vi "OP30 Indicators.vi"(8 "error in (no error)":errorcluster, 10 "Array":refnum<vi>[](array[refnum]), 11 "OUTPUT INDICATOR in":T1) -> (0 "error out":errorcluster, 3 "OUTPUT INDICATOR out":T1)   [LabVIEW 2017]
uses:
  f95f8c13-f30c-4ba5-8700-8ca84cf3f7c2.vi
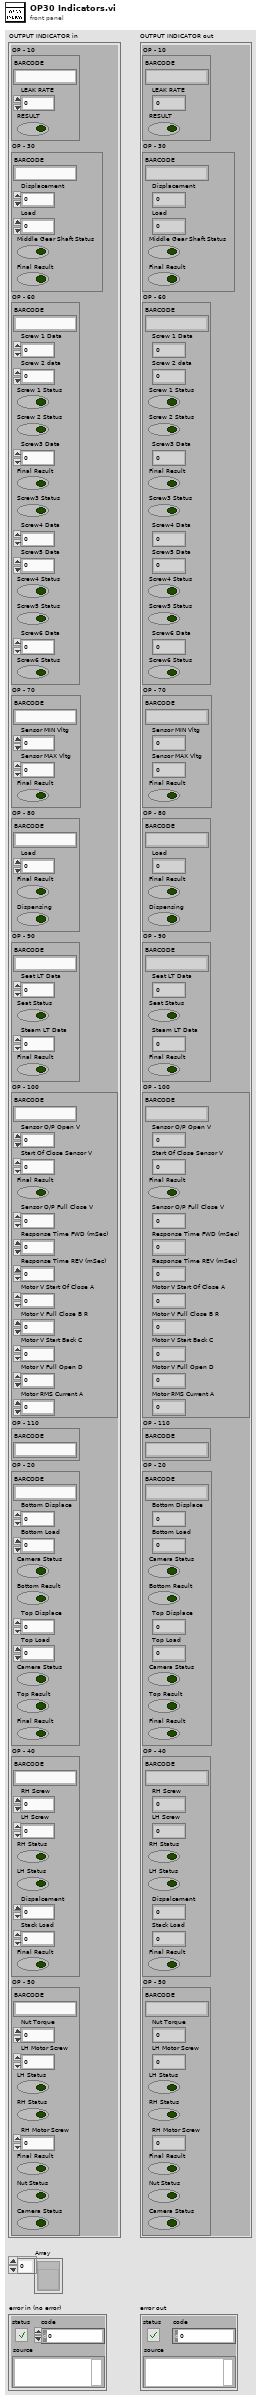
[diagram p1: front panel]
types:
  T1 = cluster{"OP - 10":cluster{"BARCODE":string, "LEAK RATE":dbl, "RESULT":bool}, "OP - 30":cluster{"BARCODE":string, "Displacement":dbl, "Load":dbl, "Middle Gear Shaft Status":bool, "Final Result":bool}, "OP - 60":cluster{"BARCODE":string, "Screw 1 Data":dbl, "Screw 2 data":dbl, "Screw 1 Status":bool, "Screw 2 Status":bool, "Screw3 Data":dbl, "Final Result":bool, "Screw3 Status":bool, "Screw4 Data":dbl, "Screw5 Data":dbl, "Screw4 Status":bool, "Screw5 Status":bool, "Screw6 Data":dbl, "Screw6 Status":bool}, "OP - 70":cluster{"BARCODE":string, "Sensor MIN Vltg":dbl, "Sensor MAX Vltg":dbl, "Final Result":bool}, "OP - 80":cluster{"BARCODE":string, "Load":dbl, "Final Result":bool, "Dispensing":bool}, "OP - 90":cluster{"BARCODE":string, "Seat LT Data":dbl, "Seat Status":bool, "Steam LT Data":dbl, "Final Result":bool}, "OP - 100":cluster{"BARCODE":string, "Sensor O/P Open V":dbl, "Start Of Close Sensor V":dbl, "Final Result":bool, "Sensor O/P Full Close V":dbl, "Response Time FWD (mSec)":dbl, "Response Time REV (mSec)":dbl, "Motor V Start Of Close A":dbl, "Motor V Full Close B R":dbl, "Motor V Start Back C":dbl, "Motor V Full Open D":dbl, "Motor RMS Current A":dbl}, "OP - 110":cluster{"BARCODE":string}, "OP - 20":cluster{"BARCODE":string, "Bottom Displace":dbl, "Bottom Load":dbl, "Camera Status":bool, "Bottom Result":bool, "Top Displace":dbl, "Top Load ":dbl, "Camera Status":bool, "Top Result":bool, "Final Result":bool}, "OP - 40":cluster{"BARCODE":string, "RH Screw":dbl, "LH Screw ":dbl, "RH Status":bool, "LH Status":bool, "Dispalcement ":dbl, "Stack Load ":dbl, "Final Result":bool}, "OP - 50":cluster{"BARCODE":string, "Nut Torque":dbl, "LH Motor Screw":dbl, "LH Status":bool, "RH Status":bool, "RH Motor Screw":dbl, "Final Result":bool, "Nut Status":bool, "Camera Status":bool}}
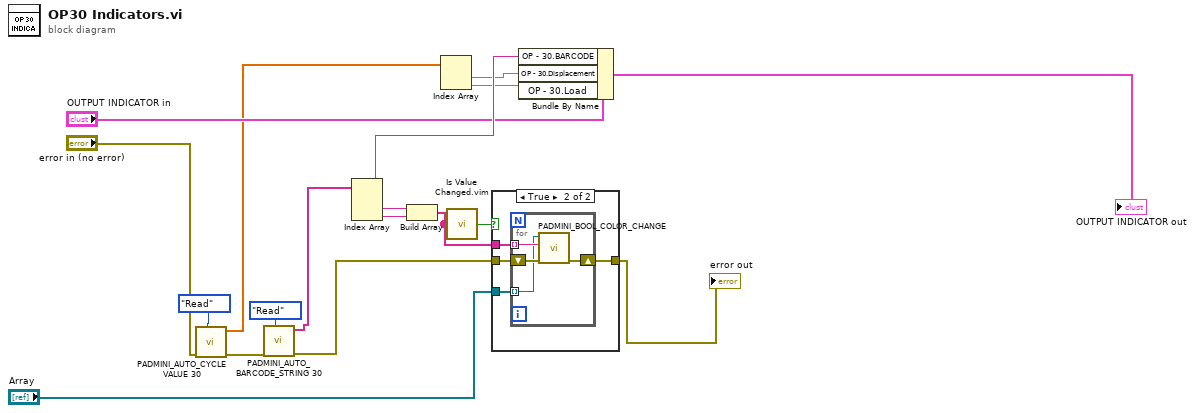
[diagram p0: block diagram]
diagram:
  n1 = call "PADMINI_AUTO_CYCLE VALUE 30.vi"("Enum"=enum16{"Read", "Write"}."Read", "error in (no error)"="error in (no error)") -> ("error out"=w7:errorcluster, "Input 2"=w3:sgl[])  [unwired: 8 in]
  n2 = call "PADMINI_AUTO_BARCODE_STRING 30.vi"("Enum"=enum16{"Read", "Write"}."Read", "error in (no error)"=w7) -> ("error out"=w14:errorcluster, "Input 2"=w13:string[])  [unwired: 8 in]
  n3 = Index Array(array=w13) -> (element #1=w15:string, element #2=w11:string, element #3=w10:string)  [unwired: 3 in]
  n4 = Build Array(w11, w10) -> (w9:string[])
  n5 = Index Array(array=w3) -> (element #1=w5:sgl, element #2=w6:sgl)  [unwired: 2 in]
  n6 = call "Is Value Changed.vim"("value"=w9) -> ("changed or first call?"=w12:bool)
  n7 = case shown="True" w12 {
    tunnel: [w19 w23] -> w18
    tunnel: w9 -> [_ w22]
    tunnel: w14 -> [w19 w21]
    tunnel: "Array" -> [_ w20]
    frame False {
    }
    frame True {
      n8 = for {
        tunnel: w22 -> [w26] mode=indexing
        shift-right: [w27] -> w23
        shift-left: w21 -> [w25]
        tunnel: w20 -> [w24] mode=indexing
        n9 = call "PADMINI_BOOL_COLOR_CHANGE.vi"("error in (no error)"=w25, "Input Result"=w26, "Boolean in"=w24) -> ("error out"=w27:errorcluster)  [unwired: 8 in]
      }
    }
  }
  "error out" <- w18
  n10 = Bundle By Name(cluster="OUTPUT INDICATOR in", "OP - 30.BARCODE"=w15, "OP - 30.Displacement"=w5, "OP - 30.Load"=w6) -> (→"OUTPUT INDICATOR out":T1)
